vi "register_events.vi"(6 "Action":T2, 7 "Events to register":T1[](array[typedef]), 8 "error in (no error)":errorcluster, 11 "BalloonNotifier in":refnum<class "BalloonNotifier.lvclass">) -> (0 "error out":errorcluster, 3 "BalloonNotifier out":refnum<class "BalloonNotifier.lvclass">)   [LabVIEW 2010, in "BalloonNotifier.lvclass"]
uses:
  BalloonNotifier.lvclass
  balloon_event_registration_actions.ctl
  balloon_events.ctl
  balloon_event_data.ctl
  ballloon_user_event_ref.ctl
  BalloonNotifier.lvclass/BalloonNotifier.ctl
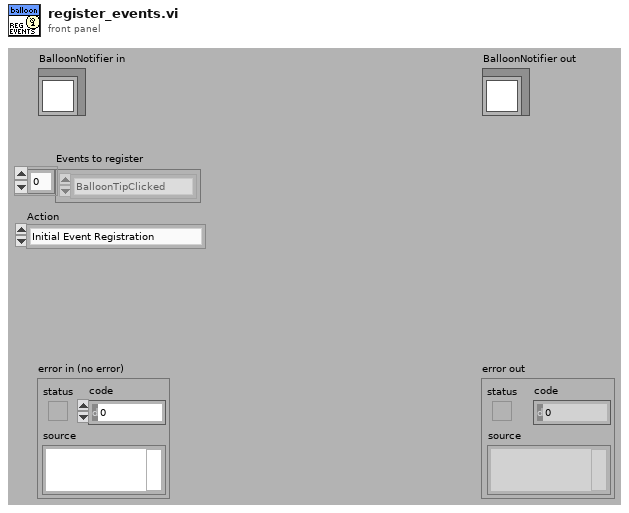
[diagram p1: front panel]
types:
  T1 = typedef "BalloonNotifier.lvclass/balloon_events.ctl" = enum16{"BalloonTipClicked", "BalloonTipClosed", "BalloonTipShown", "Click", "Disposed", "DoubleClick", "MouseClick", "MouseDoubleClick", "MouseDown", "MouseMove", "MouseUp", "MenuItemClick", "MenuItemSelect"}
  T2 = typedef "BalloonNotifier.lvclass/balloon_event_registration_actions.ctl" = enum16{"Initial Event Registration", "Add to Event Registration", "Destroy Events and Re-register"}
  T3 = typedef "BalloonNotifier.lvclass/balloon_event_data.ctl" = cluster{"NotifyIcon Event":T1, "Data String":string}
  T4 = typedef "BalloonNotifier.lvclass/ballloon_user_event_ref.ctl" = refnum<user-event>
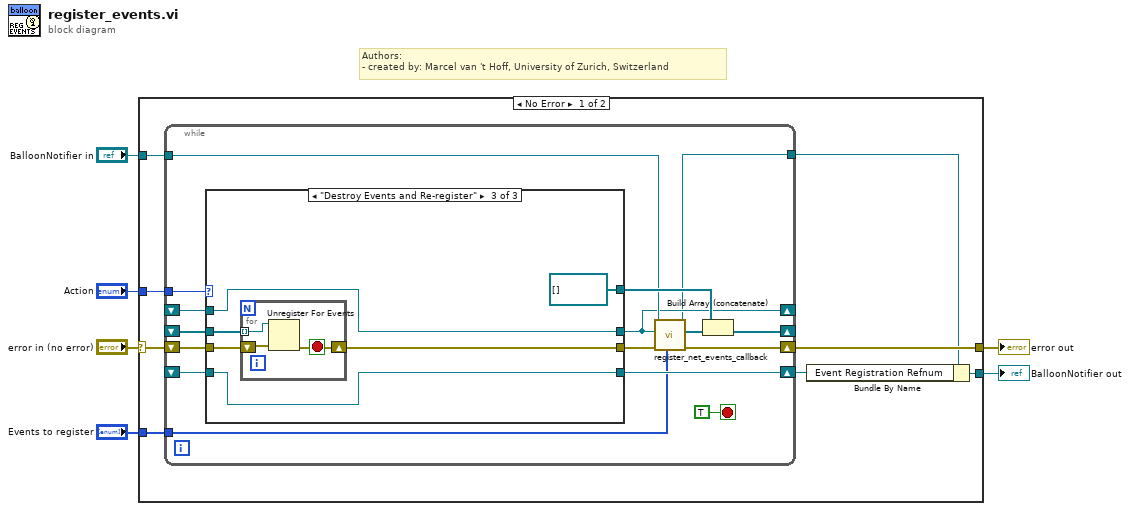
[diagram p0: block diagram]
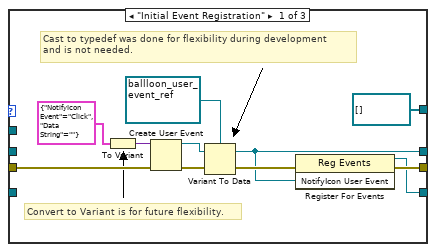
[diagram p2: hidden frame]
diagram:
  # "Authors: \n- created by: Marcel van 't Hoff, University of Zurich, Switzerland"
  n1 = case shown="No Error" "error in (no error)" {
    selector: "error in (no error)" -> [w12 w56]
    tunnel: "Events to register" -> [w14 _]
    tunnel: [w13 w56] -> w5
    tunnel: "Action" -> [w11 _]
    tunnel: "BalloonNotifier in" -> [w8 w55]
    tunnel: [w9 w55] -> w1
    frame No Error {
      n2 = while {
        tunnel: w14 -> [w19]
        tunnel: w11 -> [w27]
        shift-right: [w20] -> _
        shift-left: _ -> [w26]
        shift-right: [w30] -> w10
        shift-left: _ -> [w25]
        shift-right: [w23] -> _
        shift-left: _ -> [w24]
        shift-right: [w16] -> w13
        shift-left: w12 -> [w29]
        tunnel: w8 -> [w21]
        tunnel: [w15] -> w7
        stop <- TRUE stop-if-true
        n3 = case shown="\"Destroy Events and Re-register\"" w27 {
          tunnel: [w35 w44 w48] -> w17
          tunnel: [w34 w45 w49] -> w20
          tunnel: [w33 w43 w47] -> w30
          tunnel: w29 -> [w32 w44 w51]
          tunnel: w26 -> [_ w45 w49]
          tunnel: w25 -> [_ w43 w47]
          tunnel: w24 -> [_ w42 w50]
          tunnel: [refnum<k27>[] [] w42 refnum<k27>[] []] -> w22
          frame "Initial Event Registration" {
            # "Cast to typedef was done for flexibility during development\nand is not needed."
            # "Convert to Variant is for future flexibility."
            n4 = To Variant(anything=T3 {"NotifyIcon Event"=enum."Click", "Data String"=""} ("NotifyIcon Event Data")) -> (Variant=w39:variant)
            n5 = Create User Event(user event datatype=w39, error in=w32) -> (user event=w38:refnum<user-event>, error out=w41:errorcluster)
            n6 = Variant To Data(error in=w41, Variant=w38, type=T4 refnum ("NotifyIcon User Event")) -> (error out=w40:errorcluster, data=w34:T4)
            n7 = register-events(error in=w40, w34) -> (reference out=w33:refnum<event-registration>, error out=w35:errorcluster)  [unwired: 1 in]
          }
          frame "Add to Event Registration", Default {
          }
          frame "Destroy Events and Re-register" {
            n8 = for {
              tunnel: w50 -> [w53] mode=indexing
              shift-right: [w52] -> w48
              shift-left: w51 -> [w54]
              stop <- w52 stop-if-true
              n9 = Unregister For Events(event registration refnum=w53, error in=w54) -> (error out=w52:errorcluster)
            }
          }
        }
        n10 = call-dynamic "register_net_events_callback.vi"("Events to register"=w19, "error in (no error)"=w17, "NotifyIcon User Event Ref"=w20, "BalloonNotifier in"=w21) -> ("error out"=w16:errorcluster, ".NET event refs"=w18:refnum<k27>[], "BalloonNotifier out"=w15:refnum<class "BalloonNotifier.lvclass">)  [unwired: 5 in]
        n11 = Build Array (concatenate)(w22, w18) -> (w23:refnum<k27>[])
      }
      n12 = Bundle By Name(cluster=w7, "Event Registration Refnum"=w10) -> (w9:refnum<class "BalloonNotifier.lvclass">)
    }
    frame Error {
    }
  }
  "error out" <- w5
  "BalloonNotifier out" <- w1
